vi "RichToFlatnixnet_grpc_WriteStateRequest.vi"(5 "OutputClusterType":T1, 11 "InputCluster":T7) -> (3 "OutputCluster":T1)   [LabVIEW 2025, in "grpc-xnet_client.lvlib"]
uses:
  grpc-xnet_client.lvlib
  nixnet_grpc_WriteStateRequest.ctl
  nixnet_grpc_WriteStateRequest_state_id_enum/nixnet_grpc_WriteStateRequest_state_id_enum.lvclass
  nixnet_grpc_WriteStateValue_value/nixnet_grpc_WriteStateValue_value.lvclass
  nidevice_grpc_Session.ctl
  nixnet_grpc_WriteStateValue.ctl
  nixnet_grpc_WriteStateRequest_Flat.ctl
  nidevice_grpc_Session_Flat.ctl
  nixnet_grpc_WriteState.ctl
  nixnet_grpc_WriteStateValue_Flat.ctl
  nixnet_grpc_LinDiagnosticScheduleChangeRequest_Flat.ctl
  nixnet_grpc_LinDiagnosticSchedule.ctl
  nixnet_grpc_WriteStateRequest_state_id_enum/nixnet_grpc_WriteStateRequest_state_id_enum.lvclass/nixnet_grpc_WriteStateRequest_state_id_enum.ctl
  nixnet_grpc_WriteStateValue_value/nixnet_grpc_WriteStateValue_value.lvclass/nixnet_grpc_WriteStateValue_value.ctl
  nixnet_grpc_LinDiagnosticScheduleChangeRequest_schedule_enum/nixnet_grpc_LinDiagnosticScheduleChangeRequest_schedule_enum.lvclass/nixnet_grpc_LinDiagnosticScheduleChangeRequest_schedule_enum.ctl
  nixnet_grpc_WriteStateValue_value/Getlin_schedule_change.vi
  nixnet_grpc_WriteStateValue_value/Getflex_ray_symbol.vi
  nixnet_grpc_WriteStateValue_value/Getlin_diagnostic_schedule_change.vi
  RichToFlatnixnet_grpc_LinDiagnosticScheduleChangeRequest.vi
  nixnet_grpc_WriteStateValue_value/Getethernet_sleep.vi
  nixnet_grpc_WriteStateValue_value/Getethernet_wake.vi
  nixnet_grpc_LinDiagnosticScheduleChangeRequest_schedule_enum/Getschedule.vi
  nixnet_grpc_LinDiagnosticScheduleChangeRequest_schedule_enum/Getschedule_raw.vi
  nixnet_grpc_LinDiagnosticScheduleChangeRequest_schedule_enum/nixnet_grpc_LinDiagnosticScheduleChangeRequest_schedule_enum.lvclass
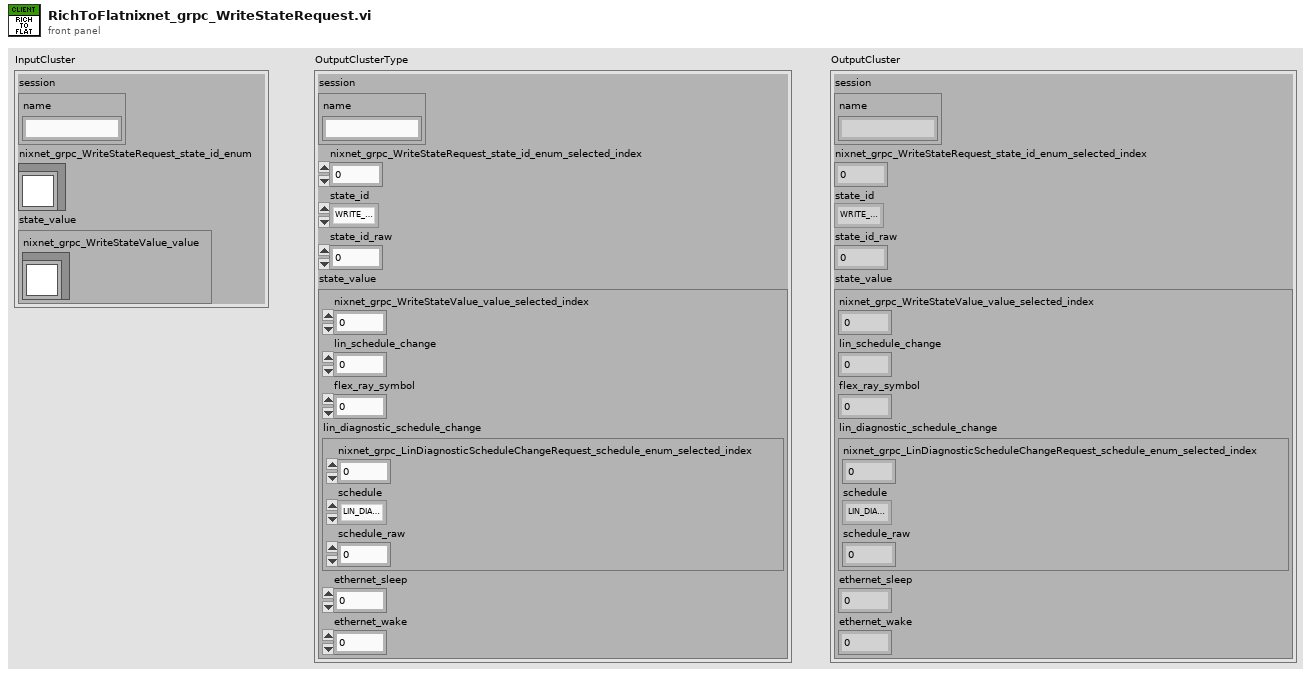
[diagram p1: front panel]
types:
  T1 = typedef "grpc-xnet_client.lvlib/nixnet_grpc_WriteStateRequest_Flat.ctl" = cluster{"session":T2, "nixnet_grpc_WriteStateRequest_state_id_enum_selected_index":i32, "state_id":T3, "state_id_raw":u32, "state_value":T4}
  T2 = typedef "grpc-xnet_client.lvlib/nidevice_grpc_Session_Flat.ctl" = cluster{"name":string}
  T3 = typedef "grpc-xnet_client.lvlib/nixnet_grpc_WriteState.ctl" = enum32{"WRITE_STATE_UNSPECIFIED", "WRITE_STATE_LIN_SCHEDULE_CHANGE", "WRITE_STATE_LIN_DIAGNOSTIC_SCHEDULE_CHANGE", "WRITE_STATE_FLEX_RAY_SYMBOL", "WRITE_STATE_ETHERNET_SLEEP", "WRITE_STATE_ETHERNET_WAKE"}
  T4 = typedef "grpc-xnet_client.lvlib/nixnet_grpc_WriteStateValue_Flat.ctl" = cluster{"nixnet_grpc_WriteStateValue_value_selected_index":i32, "lin_schedule_change":u32, "flex_ray_symbol":u32, "lin_diagnostic_schedule_change":T5, "ethernet_sleep":u32, "ethernet_wake":u32}
  T5 = typedef "grpc-xnet_client.lvlib/nixnet_grpc_LinDiagnosticScheduleChangeRequest_Flat.ctl" = cluster{"nixnet_grpc_LinDiagnosticScheduleChangeRequest_schedule_enum_selected_index":i32, "schedule":T6, "schedule_raw":u32}
  T6 = typedef "grpc-xnet_client.lvlib/nixnet_grpc_LinDiagnosticSchedule.ctl" = enum32{"LIN_DIAGNOSTIC_SCHEDULE_NULL", "LIN_DIAGNOSTIC_SCHEDULE_MASTER_REQ", "LIN_DIAGNOSTIC_SCHEDULE_SLAVE_RESP"}
  T7 = typedef "grpc-xnet_client.lvlib/nixnet_grpc_WriteStateRequest.ctl" = cluster{"session":T8, "nixnet_grpc_WriteStateRequest_state_id_enum":refnum<class "nixnet_grpc_WriteStateRequest_state_id_enum.lvclass">, "state_value":T9}
  T8 = typedef "grpc-xnet_client.lvlib/nidevice_grpc_Session.ctl" = cluster{"name":string}
  T9 = typedef "grpc-xnet_client.lvlib/nixnet_grpc_WriteStateValue.ctl" = cluster{"nixnet_grpc_WriteStateValue_value":refnum<class "nixnet_grpc_WriteStateValue_value.lvclass">}
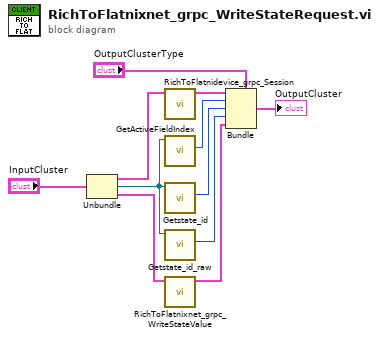
[diagram p0: block diagram]
diagram:
  n1 = Unbundle "Unbundle"("InputCluster") -> ("session"=w8:T8, "nixnet_grpc_WriteStateRequest_state_id_enum"=w6:refnum<class "nixnet_grpc_WriteStateRequest_state_id_enum.lvclass">, "state_value"=w2:T9)
  n2 = call "RichToFlatnidevice_grpc_Session.vi"("InputCluster"=w8) -> ("OutputCluster"=w7:T2)  [unwired: 10 in]
  n3 = call "GetActiveFieldIndex.vi"("OneOfTemplate in"=w6) -> ("Active Field Index"=w5:i32)  [unwired: 8 in, 2 out]
  n4 = call "Getstate_id.vi"("OneOfTemplate in"=w6) -> ("Get_Val"=w4:T3)  [unwired: 8 in, 2 out]
  n5 = call "Getstate_id_raw.vi"("OneOfTemplate in"=w6) -> ("Get_Val"=w3:u32)  [unwired: 8 in, 2 out]
  n6 = call "RichToFlatnixnet_grpc_WriteStateValue.vi"("InputCluster"=w2) -> ("OutputCluster"=w1:T4)  [unwired: 10 in]
  n7 = Bundle "Bundle"(cluster="OutputClusterType", "session"=w7, "nixnet_grpc_WriteStateRequest_state_id_enum_selected_index"=w5, "state_id"=w4, "state_id_raw"=w3, "state_value"=w1) -> (→"OutputCluster":T1)
